vi "ZenAnalytic_API.vi"() -> ()   [LabVIEW 2015]
panel:
  in  "Graph Refference's":T1
  in  "GraphRefference":bool=TRUE
  in  "String 22":string="GraphRefferenceForPrint"
  in  "Inter Actor event data":cluster{"State Name":string, "Data":variant}={"State Name"="Init", "Data"=variant}
  in  "Back":bool=TRUE
  in  "String 16":string="Back"
  in  "String 21":string="StatisticalData"
  in  "StatisticalData":bool=TRUE
  in  "Pause":bool=TRUE
  in  "Statistical Data":string[][](array[string])=[["", "Measurement1", "Measurement2", "Measurement3", "Measurement N"], ["Mean", "", "", "", ""], ["Standard Deviation", "", "", "", ""], ["Variance", "", "", "", ""], ["Cp", "", "", "", ""], ["CpK", "", "", "", ""]]
  in  "Stop":bool=TRUE
  in  "Analytics":bool=TRUE
  in  "ResultCluster":T2
  in  "Initialization Values":T3
  in  "String 19":string="Stop"
  in  "String 15":string="Pause"
  in  "String 5":string="Analytics"
  in  "String 3":string="ResultData"
  in  "String 2":string="Init"
  # "Intra Actor Communication APIs:"
  # "This is a User Event which is a part of ZenAnalytics Actor and is used to Recieve Data from State Machine"
  # "Event Data: Cluster of String(Typr Of Data) and Variant(Data)"
  # "Convert the data to variant and then feed it into the event data cluster."
  # "Operation"
  # "State"
  # "Data"
  # "Once the part selection is done"
  # "Inspection Result Data"
  # "Note : \n\nThere is VI named Output_ZA.vi\nWhere state machine can recieve analytics info\n\nSuch as \nActorInfo - which has analytics UI refference\nStatInfo - Statistical parameters for cumulative data\nGraphInfo - Graph Refference for print \n\nCan Edit Analytics GUI named UserInterface_ZA.vi"
  # "Analytics ButtonPress Event"
  # "Pause ButtonPress Event"
  # "Back ButtonPress Event"
  # "Stop ButtonPress Event"
  # "Recieve Statistical Data from Analytics"
  # "Recieve Graphs Refference from Analytics for Print"
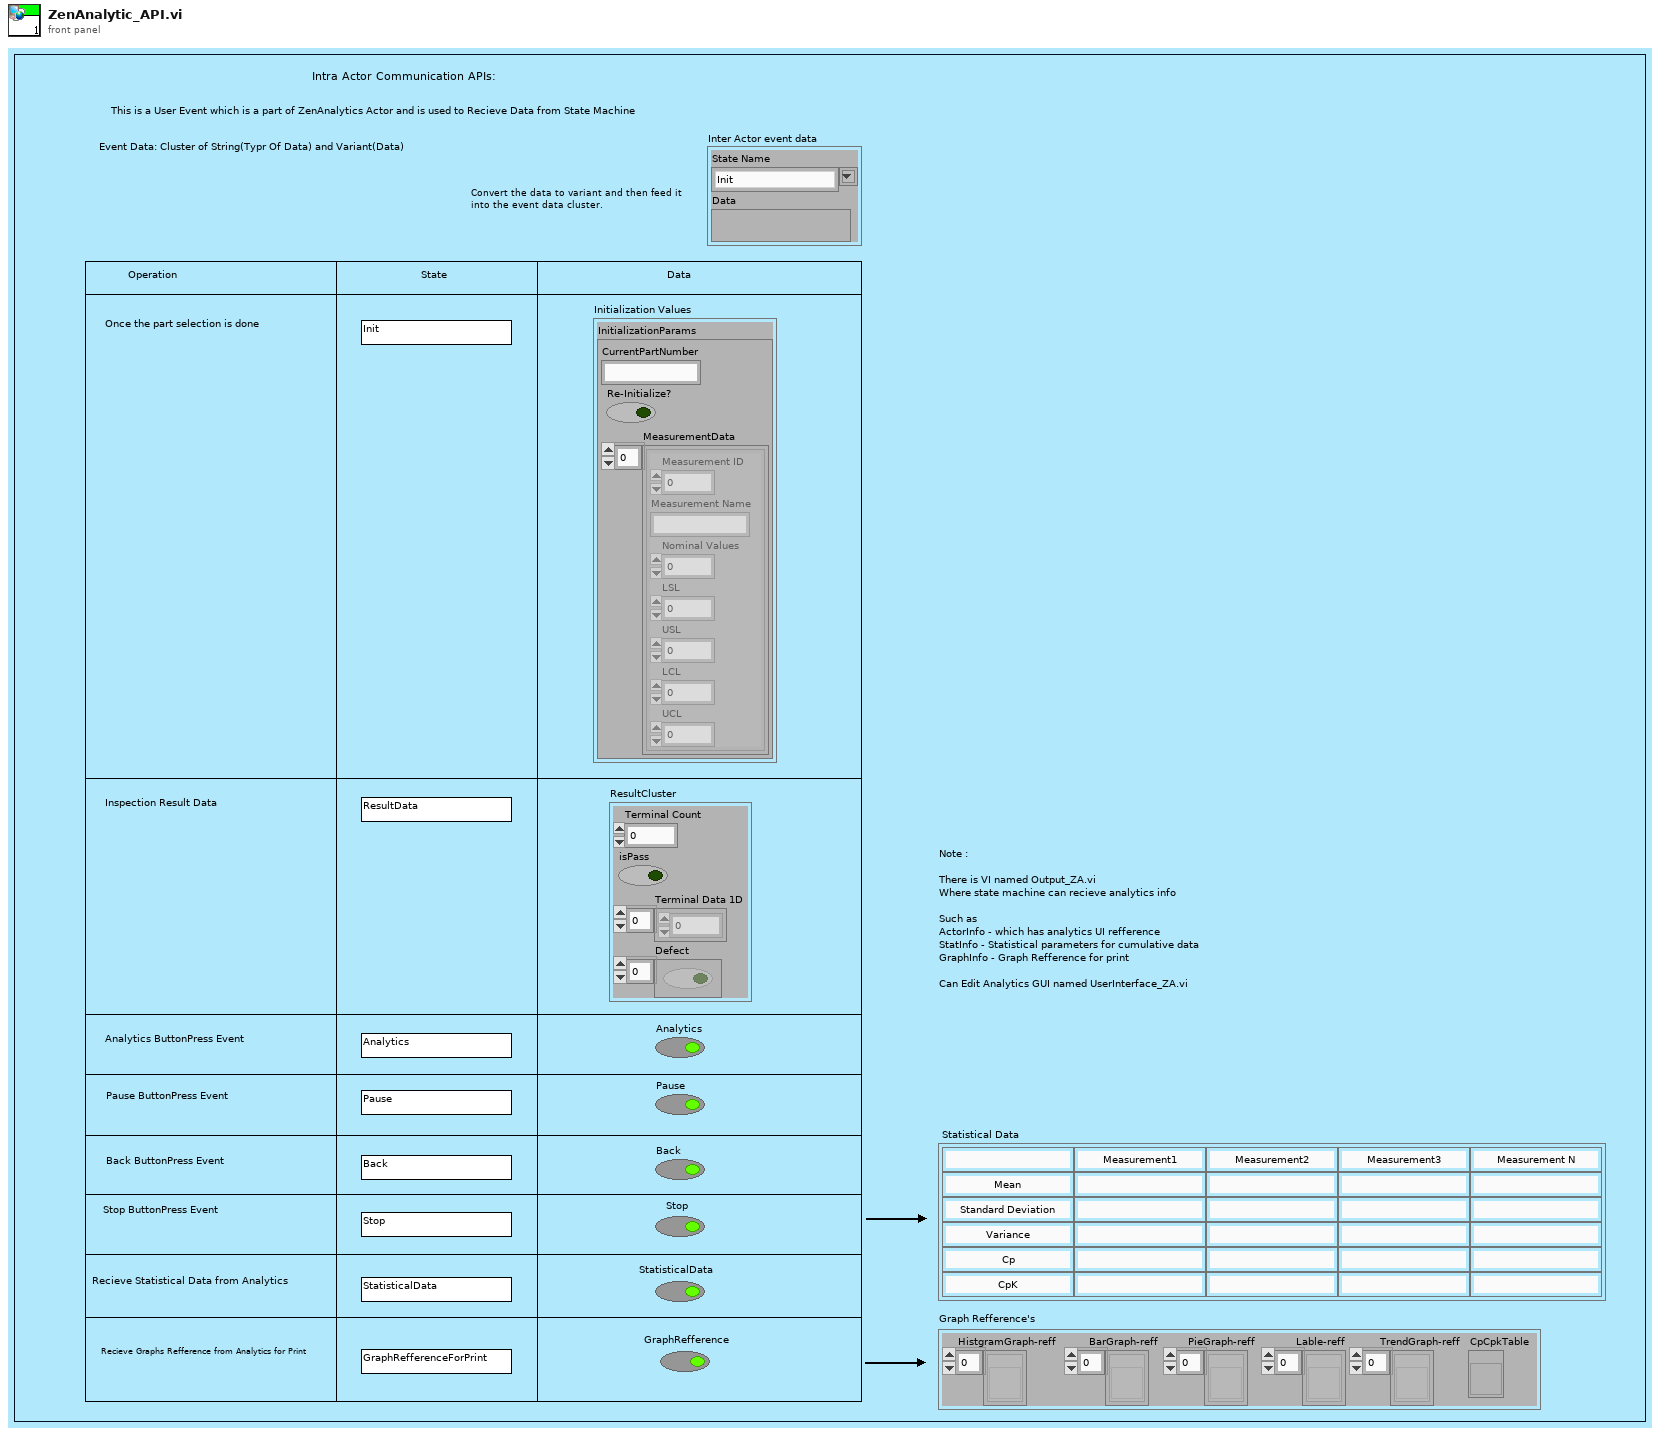
[diagram p1: front panel]
types:
  T1 = cluster{"HistgramGraph-reff":refnum<vi>[], "BarGraph-reff":refnum<vi>[], "PieGraph-reff":refnum<vi>[], "Lable-reff":refnum<vi>[], "TrendGraph-reff":refnum<vi>[], "CpCpkTable":refnum<vi>}
  T2 = cluster{"Terminal Count":u32, "isPass":bool, "Terminal Data 1D":dbl[], "Defect":bool[]}
  T3 = cluster{"InitializationParams":cluster{"CurrentPartNumber":string, "Re-Initialize?":bool, "MeasurementData":cluster{"Measurement ID":i32, "Measurement Name":string, "Nominal Values":dbl, "LSL":dbl, "USL":dbl, "LCL":dbl, "UCL":dbl}[]}}
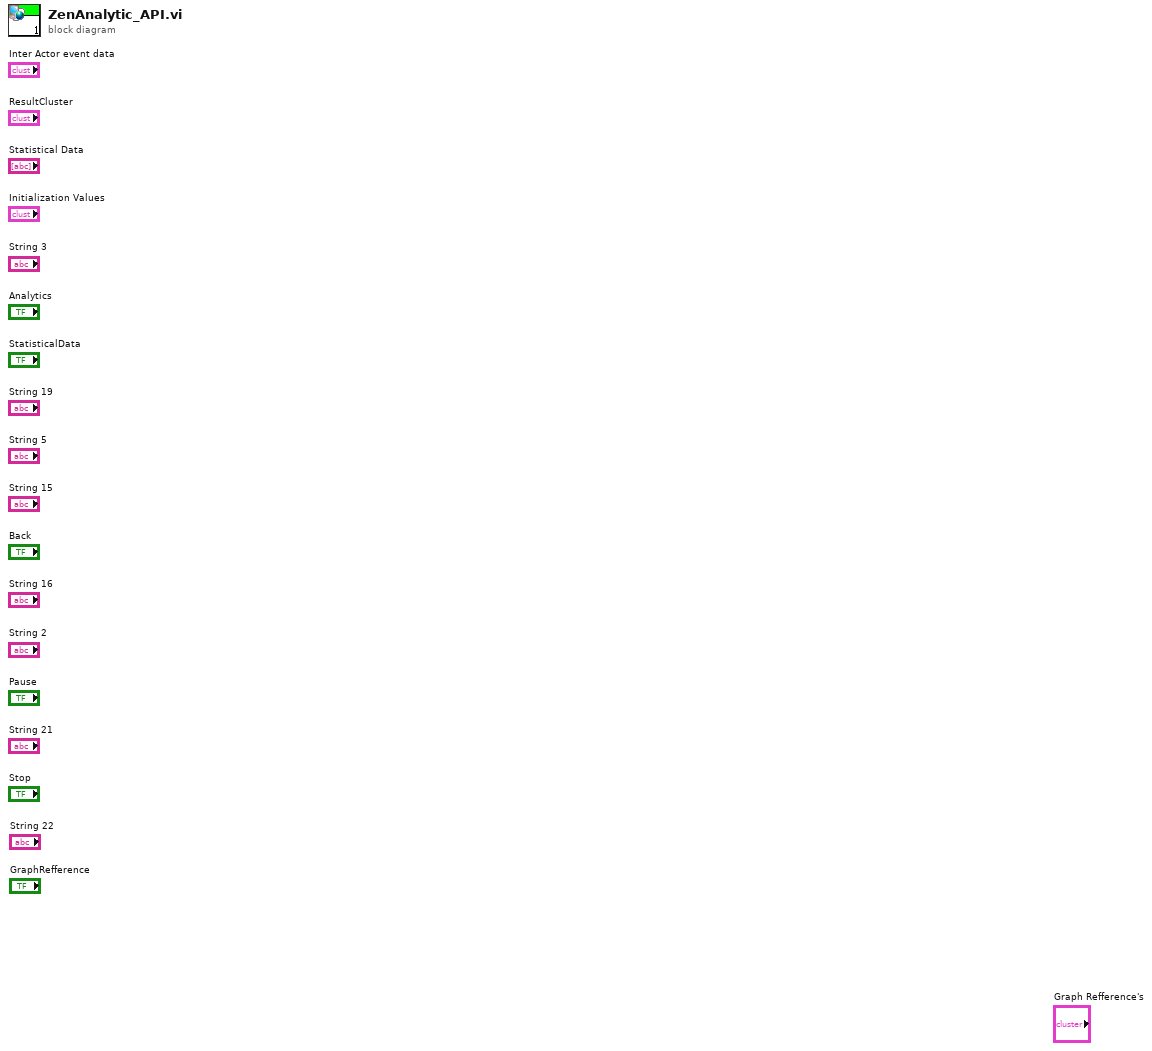
[diagram p0: block diagram]
diagram:
